vi "GetNextFocus.vi"(8 "error in (no error)":errorcluster, 11 "TelFocus in":refnum<class "TelFocus.lvclass">) -> (0 "error out":errorcluster, 3 "TelFocus out":refnum<class "TelFocus.lvclass">)   [LabVIEW 2018, in "TelFocus.lvclass"]
uses:
  TelFocus.lvclass
  TelFocus.lvclass/TelFocus.ctl
  SecMirror/SecMirror.lvclass
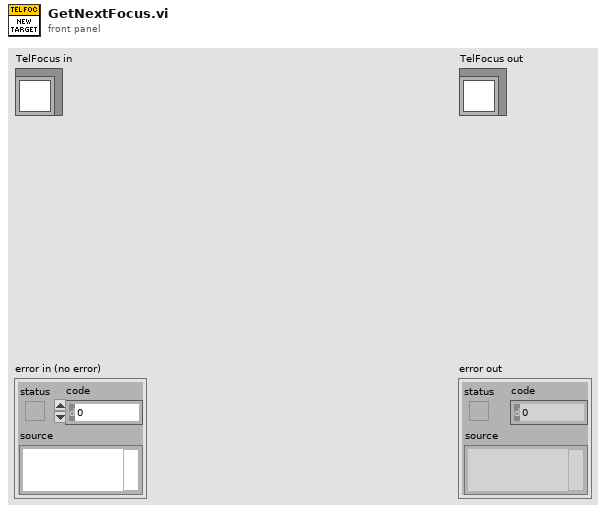
[diagram p1: front panel]
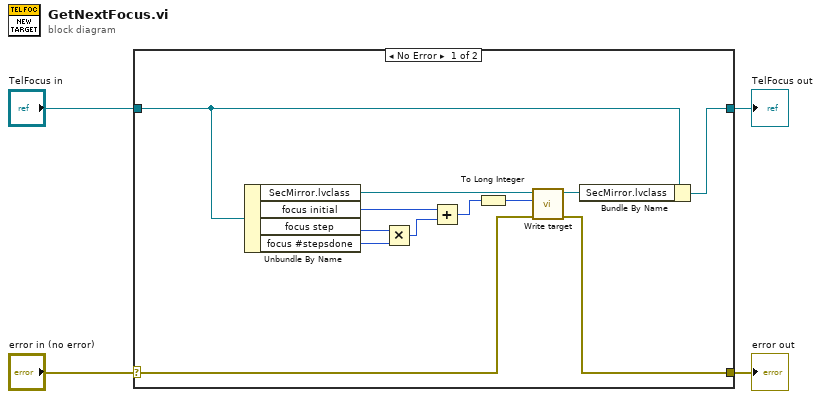
[diagram p0: block diagram]
diagram:
  n1 = case shown="No Error" "error in (no error)" {
    selector: "error in (no error)" -> [w7 w18]
    tunnel: [w6 w18] -> w3
    tunnel: [w15 w17] -> w1
    tunnel: "TelFocus in" -> [w16 w17]
    frame No Error {
      n2 = Unbundle By Name(w16) -> ("SecMirror.lvclass"=w13:refnum<class "SecMirror.lvclass">, "focus initial"=w11:i32, "focus step"=w10:i32, "focus #stepsdone"=w9:u32)
      n3 = Multiply(x=w10, y=w9) -> (x*y=w12:u32)
      n4 = Add(x=w11, y=w12) -> (x+y=w8:u32)
      n5 = To Long Integer(number=w8) -> (32bit integer=w5:i32)
      n6 = call-dynamic "Write target.vi"("error in (no error)"=w7, "target"=w5, "SecMirror in"=w13) -> ("error out"=w6:errorcluster, "SecMirror out"=w14:refnum<class "SecMirror.lvclass">)  [unwired: 7 in]
      n7 = Bundle By Name(cluster=w16, "SecMirror.lvclass"=w14) -> (w15:refnum<class "TelFocus.lvclass">)
    }
    frame Error {
    }
  }
  "error out" <- w3
  "TelFocus out" <- w1
